vi "Channel to Bit.vi"(4 "dst byte order":T3(ring), 5 "src channel descriptor":T1 {"buffer offset" format="%d bytes"}, 6 "src byte order":T3(ring), 8 "error in (no error)":errorcluster, 9 "channel count":u64, 10 "dst buffer in":string, 11 "src buffer in":string) -> (0 "error out":errorcluster, 2 "dst buffer out":string, 3 "src buffer out":string)   [LabVIEW 2017, in "DSF Core.lvlib" / "Buffer Converter.lvclass"]
uses:
  Buffer Converter.lvclass
  Channel Descriptor.ctl
  Typedefs/DSF Data Type.ctl
  Clear Bit.vi
  Buffer/Buffer.lvclass
  DSF Core.lvlib
panel:
  in  "dst bit offset":u64 format="%d bits"
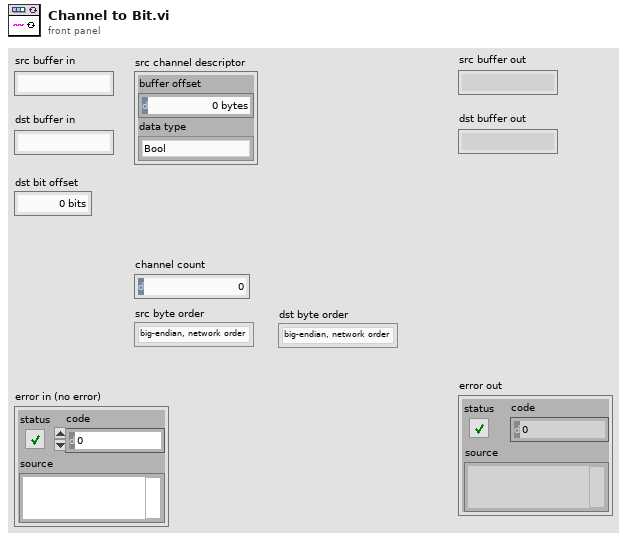
[diagram p1: front panel]
types:
  T1 = typedef "DSF Core.lvlib/Buffer.lvclass/Channel Descriptor.ctl" = cluster{"buffer offset":u64, "data type":T2}
  T2 = typedef "DSF Core.lvlib/DSF Data Type.ctl" = enum8{"Bool", "SGL", "DBL", "I8", "I16", "I32", "I64", "U8", "U16", "U32", "U64"}
  T3 = enum16{"big-endian, network order", "native, host order", "little-endian"}
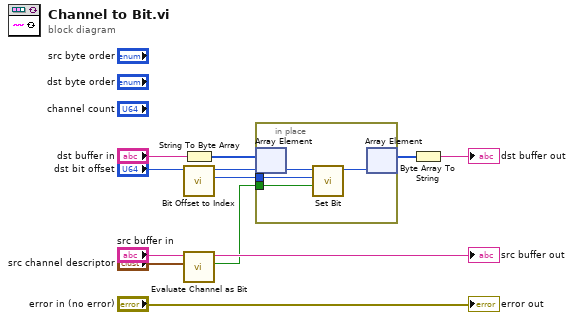
[diagram p0: block diagram]
diagram:
  n1 = String To Byte Array(string="dst buffer in") -> (unsigned byte array=w8:u8[])
  n2 = call "Bit Offset to Index.vi"("bit offset"="dst bit offset") -> ("bit index"=w6:u8, "byte offset"=w7:u64)  [unwired: 9 in]
  n3 = call "Evaluate Channel as Bit.vi"("channel descriptor"="src channel descriptor", "buffer in"="src buffer in") -> ("bit"=w1:bool, "buffer out"=→"src buffer out":string)  [unwired: 8 in]
  n4 = in-place {
    in-place-border: w6 -> [w14]
    in-place-border: w1 -> [w13]
    n5 = in-place-array #1(w8, w7) -> (w16:u8)
    n6 = call "Set Bit.vi"("bit value"=w13, "bit index"=w14, "value in"=w16) -> ("value out"=w15:u8)  [unwired: 8 in]
    n7 = in-place-array #1(w15) -> (w11:u8[])  [unwired: 1 out]
  }
  n8 = Byte Array To String(unsigned byte array=w11) -> (string=→"dst buffer out":string)
  "error out" <- "error in (no error)"
